vi "Comando_Enet_1.vi"(4 "String Enviado Canal 0":string) -> (0 "Erro Canal 1":bool, 1 "String  Recebido Canal 0":string)   [LabVIEW 2018]
uses:
  Global_Telescopio.vi
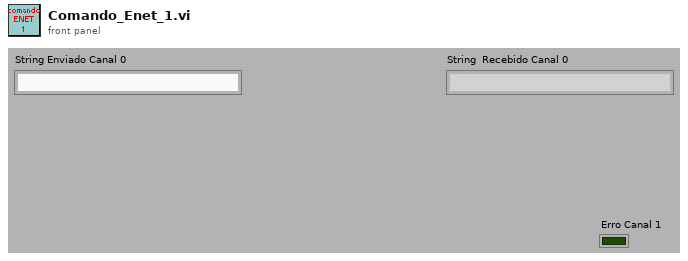
[diagram p1: front panel]
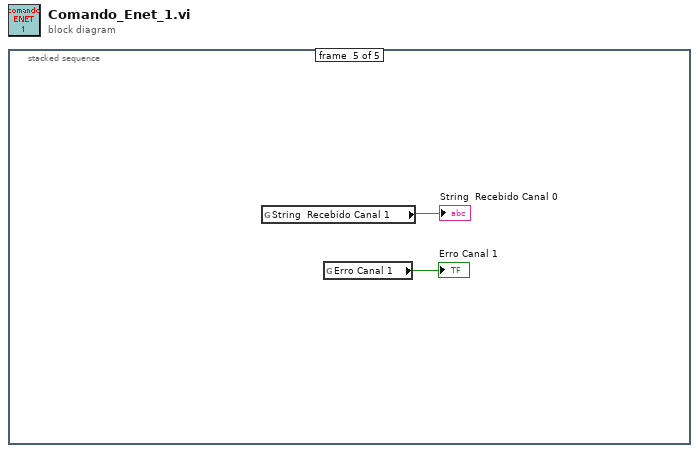
[diagram p0: block diagram]
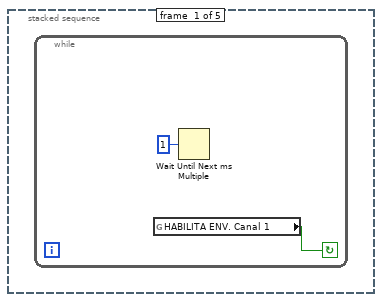
[diagram p2: hidden frame]
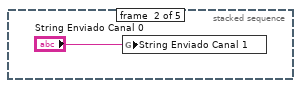
[diagram p3: hidden frame]
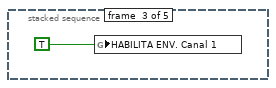
[diagram p4: hidden frame]
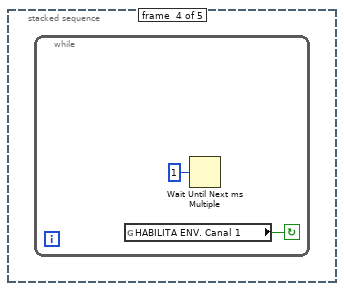
[diagram p5: hidden frame]
diagram:
  n1 = stacked-sequence {
    frame #0 {
      n2 = while {
        stop <- w2 continue-if-true
        n3 = global read "Global_Telescopio.vi" "HABILITA ENV. Canal 1"() -> (w2:bool)
        n4 = Wait Until Next ms Multiple(millisecond multiple=u32 1) -> ()  [unwired: 1 out]
      }
    }
    frame #1 {
      n5 = global write "Global_Telescopio.vi" "String Enviado Canal 1"("String Enviado Canal 0") -> ()
    }
    frame #2 {
      n6 = global write "Global_Telescopio.vi" "HABILITA ENV. Canal 1"(TRUE ("HABILITA ENV. Canal 0")) -> ()
    }
    frame #3 {
      n7 = while {
        stop <- w6 continue-if-true
        n8 = global read "Global_Telescopio.vi" "HABILITA ENV. Canal 1"() -> (w6:bool)
        n9 = Wait Until Next ms Multiple(millisecond multiple=u32 1) -> ()  [unwired: 1 out]
      }
    }
    frame #4 {
      n10 = global read "Global_Telescopio.vi" "String  Recebido Canal 1"() -> (→"String  Recebido Canal 0":string)
      n11 = global read "Global_Telescopio.vi" "Erro Canal 1"() -> (→"Erro Canal 1":bool)
    }
  }
